vi "Barycenter2D.vi"(0 "Coord Y":dbl[][](array[numeric]) format="%.2f", 3 "Coord X":dbl[][](array[numeric]) format="%.2f", 4 "Image":dbl[][](array[numeric]) format="%.2f") -> (2 "Bary Y":dbl format="%.2f", 5 "Bary X":dbl format="%.2f")   [LabVIEW 2009]
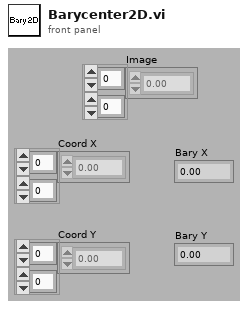
[diagram p1: front panel]
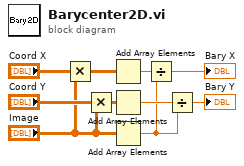
[diagram p0: block diagram]
diagram:
  n1 = Multiply(x="Coord X", y="Image") -> (x*y=w6:dbl[][])
  n2 = Multiply(x="Coord Y", y="Image") -> (x*y=w4:dbl[][])
  n3 = Add Array Elements(numeric array=w6) -> (sum=w9:dbl)
  n4 = Add Array Elements(numeric array=w4) -> (sum=w3:dbl)
  n5 = Add Array Elements(numeric array="Image") -> (sum=w2:dbl)
  n6 = Divide(x=w9, y=w2) -> (x/y=→"Bary X":dbl)
  n7 = Divide(x=w3, y=w2) -> (x/y=→"Bary Y":dbl)
